vi "ContextHelp Editor.vi"(6 "Variant in":variant, 7 "Shift Pressed?":bool, 8 "error in (no error)":errorcluster, 10 "QD Combo Box Ref":refnum<vi>, 11 "QD Launch VI Ref":refnum<vi>) -> (0 "error out":errorcluster, 4 "Variant out":variant)   [LabVIEW 2020, in "ContextHelpEditor.lvlib"]
doc: "Edit context help documentation of VIs and Typedefs easily.\nAn editor will be opened, which allows editing the documentation of the VI and all controls on the connector pane. This documentation will later be shown in the context help menu\n\nDefault Shortcut - [H]"
uses:
  _ContextHelp Editor/ContextHelpEditor.lvlib
panel:
  # "Do not change the connector pane of this VI.\n\nSee the block diagram for directions on how to use this template."
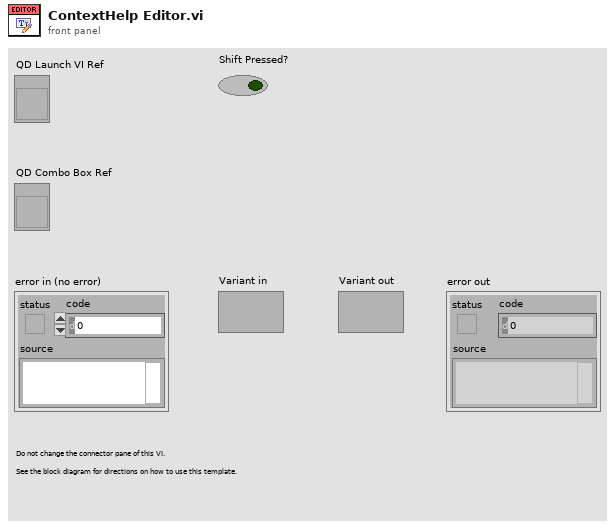
[diagram p1: front panel]
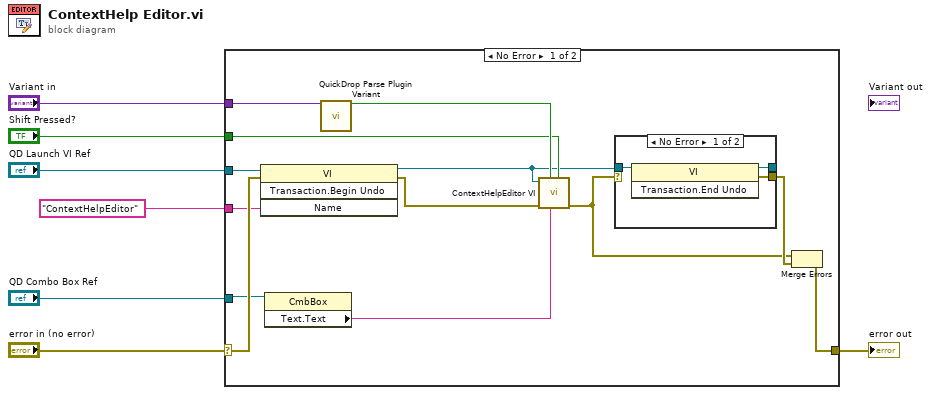
[diagram p0: block diagram]
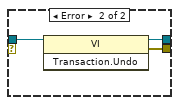
[diagram p2: hidden frame]
diagram:
  n1 = case shown="No Error" "error in (no error)" {
    selector: "error in (no error)" -> [w19 w27]
    tunnel: [w13 w27] -> w1
    tunnel: "Variant in" -> [w20 _]
    tunnel: "QD Launch VI Ref" -> [w17 _]
    tunnel: "ContextHelpEditor" ("Undo Name") -> [w18 _]
    tunnel: "Shift Pressed?" -> [w9 _]
    tunnel: "QD Combo Box Ref" -> [w14 _]
    frame No Error {
      n2 = invoke class="VI" method="Transaction.Begin Undo"(reference=w17, error in=w19, "Name"=w18) -> (reference out=w8:refnum<vi>, error out=w15:errorcluster)  [unwired: 1 in, 2 out]
      n3 = property class="CmbBox"(reference=w14) -> ("Text.Text"=w10:string)  [unwired: 1 in, 2 out]
      n4 = call <vilib>:"QuickDrop Parse Plugin Variant.vi"("QDKS Variant in"=w20) -> ("QD Launch VI Panel?"=w11:bool)  [unwired: 12 in, 2 out]
      n5 = call "ContextHelpEditor VI.vi"("Shift Pressed?"=w9, "ComboBox Text"=w10, "Executed on Frontpanel?"=w11, "error in (no error)"=w15, "VI Ref"=w8) -> ("error out"=w12:errorcluster)  [unwired: 6 in]
      n6 = case shown="No Error" w12 {
        tunnel: [w23 w26] -> w16
        tunnel: [w22 w25] -> _
        tunnel: w8 -> [w21 w24]
        frame No Error {
          n7 = invoke class="VI" method="Transaction.End Undo"(reference=w21) -> (reference out=w22:refnum<vi>, error out=w23:errorcluster)  [unwired: 2 in, 1 out]
        }
        frame Error {
          n8 = invoke class="VI" method="Transaction.Undo"(reference=w24) -> (reference out=w25:refnum<vi>, error out=w26:errorcluster)  [unwired: 2 in, 1 out]
        }
      }
      n9 = Merge Errors(w12, w16) -> (w13:errorcluster)
    }
    frame Error {
    }
  }
  "error out" <- w1
